vi "Dlg-New-Portfolio.vi"(8 "error in (no error)":errorcluster) -> (0 "error out":errorcluster)   [LabVIEW 2012]
uses:
  PortFolio/Portfolio.lvclass
panel:
  out "Portfolio out":refnum<class "Portfolio.lvclass">
  in  "Portfolio in":refnum<class "Portfolio.lvclass">
  in  "Cancel Button":bool
  in  "OK Button":bool
  in  "Help":bool
  # "Nouveau Portefeuille"
  # "Print Options"
  # "Save Options"
  # "When saving multiple files"
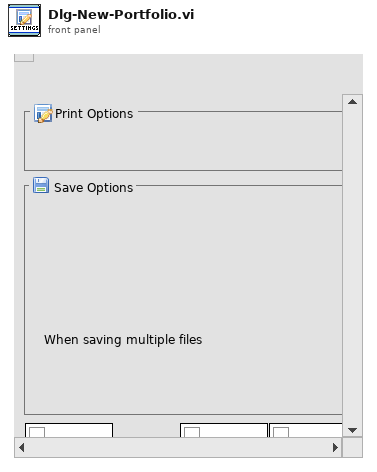
[diagram p1: front panel]
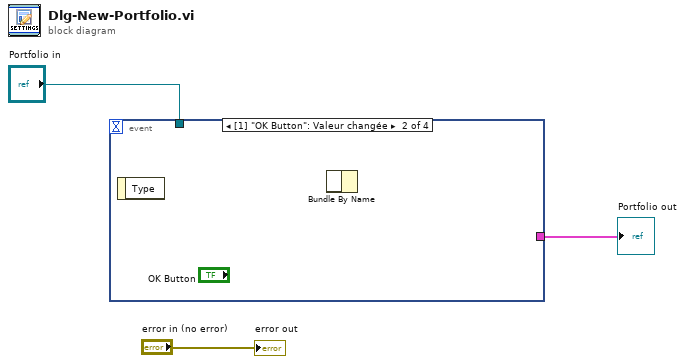
[diagram p0: block diagram]
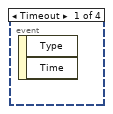
[diagram p2: hidden frame]
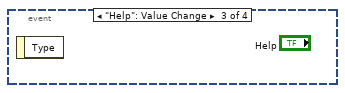
[diagram p3: hidden frame]
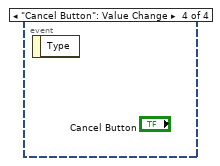
[diagram p4: hidden frame]
diagram:
  n1 = event shown="[1] \"OK Button\": Valeur changée" {
    selector: _ -> [_ _ _ _]
    dyn-events: _ -> [_ _ _ _]
    timeout: _ -> [_ _ _ _]
    tunnel: [_ _ _ _] -> w2
    tunnel: "Portfolio in" -> [_ _ _ _]
    event Timeout {
      n2 = event-data() -> ()  [unwired: 1 in, 2 out]
    }
    event "OK Button": Value Change {
      n3 = event-data() -> ()  [unwired: 1 in, 1 out]
      n4 = Bundle By Name() -> ()  [unwired: 2 in, 1 out]
    }
    event "Help": Value Change {
      n5 = event-data() -> ()  [unwired: 1 in, 1 out]
    }
    event "Cancel Button": Value Change {
      n6 = event-data() -> ()  [unwired: 1 in, 1 out]
    }
  }
  "Portfolio out" <- w2
  "error out" <- "error in (no error)"
